vi "original.vi"() -> ()   [LabVIEW 2015, in "blog-lv-interface-prototype.lvlib"]
uses:
  blog-lv-interface-prototype.lvlib
panel:
  in  "configure_build":bool
  in  "load_class":bool
  in  "dependencies":bool
  out "progress":dbl(slide) scale=0.0..100.0 scale format="%#_6f"
  in  "post":bool
  in  "cancel":bool
  in  "exit":bool
  in  "start":bool
  in  "build":bool
  in  "open_dist_folder":bool
  in  "configure":bool
  in  "select_project":bool
  in  "version":string caption="Version"
  out "commit_hash":string caption="Git Commit Hash"
  out "status":string caption="Status"
  out "project_file":string caption="Project"
  in  "error in (no error)":errorcluster
  out "error out":errorcluster
  in  "tree":string[](tree)
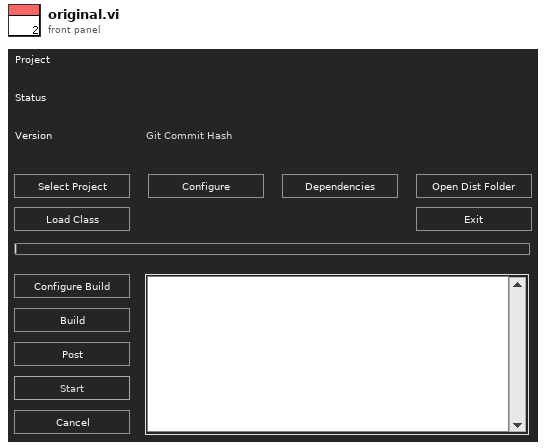
[diagram p1: front panel]
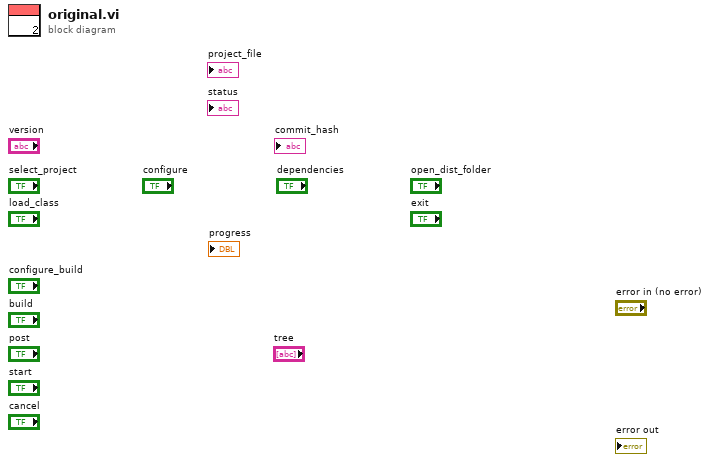
[diagram p0: block diagram]
diagram:
